vi "Read Sender.vi"(11 "Debug Data In":refnum<class "Debug Data.lvclass">) -> (2 "Sender":string, 3 "Debug Data Out":refnum<class "Debug Data.lvclass">)   [LabVIEW 2020, in "Debug Data.lvclass"]
uses:
  Debug Data.lvclass
  Debug Data.lvclass/Debug Data.ctl
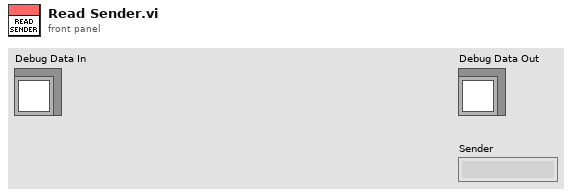
[diagram p1: front panel]
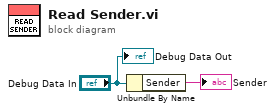
[diagram p0: block diagram]
diagram:
  n1 = Unbundle By Name("Debug Data In") -> ("Sender"=→"Sender":string)
  "Debug Data Out" <- "Debug Data In"
